vi "Router - Initial Handshaking.vi"(8 "error in (no error)":errorcluster, 11 "Router Data In":T1) -> (0 "error out":errorcluster, 3 "Router Data Out":T1)   [LabVIEW 2016, in "PXImc Router.lvlib"]
uses:
  PXImc Router.lvlib
  Controls/Router - Configuration.ctl
  Controls/Router/Node Block R-W Properties.ctl
  Controls/Router/Block Properties.ctl
  Controls/Router/Router - PXImc Properties.ctl
  Controls/Router/Router - PXImc Card Properties.ctl
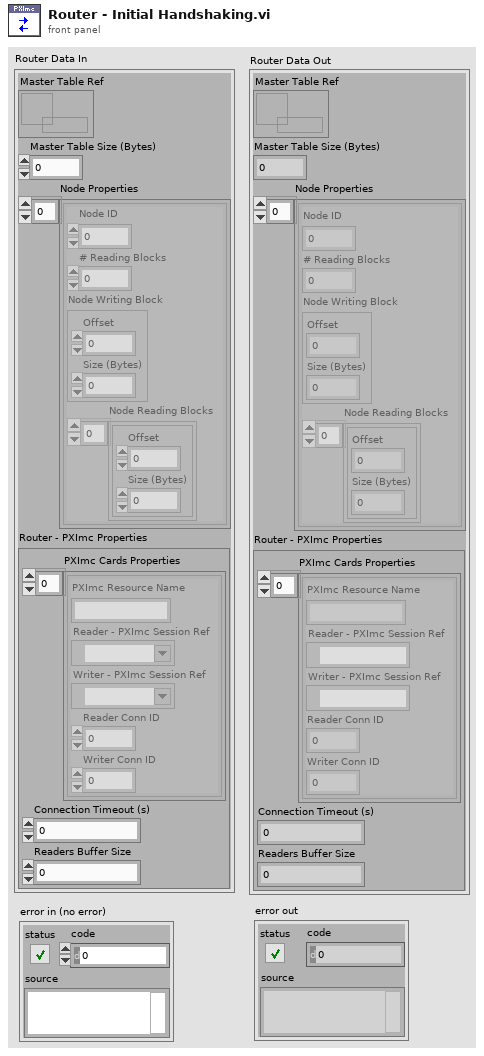
[diagram p1: front panel]
types:
  T1 = typedef "PXImc Router.lvlib/Router - Configuration.ctl" = cluster{"Master Table Ref":refnum<data-value>, "Master Table Size (Bytes)":u32, "Node Properties":T2[], "Router - PXImc Properties":T4}
  T2 = typedef "PXImc Router.lvlib/Node Block R-W Properties.ctl" = cluster{"Node ID":u32, "# Reading Blocks":u32, "Node Writing Block":T3, "Node Reading Blocks":T3[]}
  T3 = typedef "PXImc Router.lvlib/Block Properties.ctl" = cluster{"Offset":u32, "Size (Bytes)":u32}
  T4 = typedef "PXImc Router.lvlib/Router - PXImc Properties.ctl" = cluster{"PXImc Cards Properties":T5[], "Connection Timeout (s)":dbl, "Readers Buffer Size":u64}
  T5 = typedef "PXImc Router.lvlib/Router - PXImc Card Properties.ctl" = cluster{"PXImc Resource Name":string, "Reader - PXImc Session Ref":refnum<k21>, "Writer - PXImc Session Ref":refnum<k21>, "Reader Conn ID":u16, "Writer Conn ID":u16}
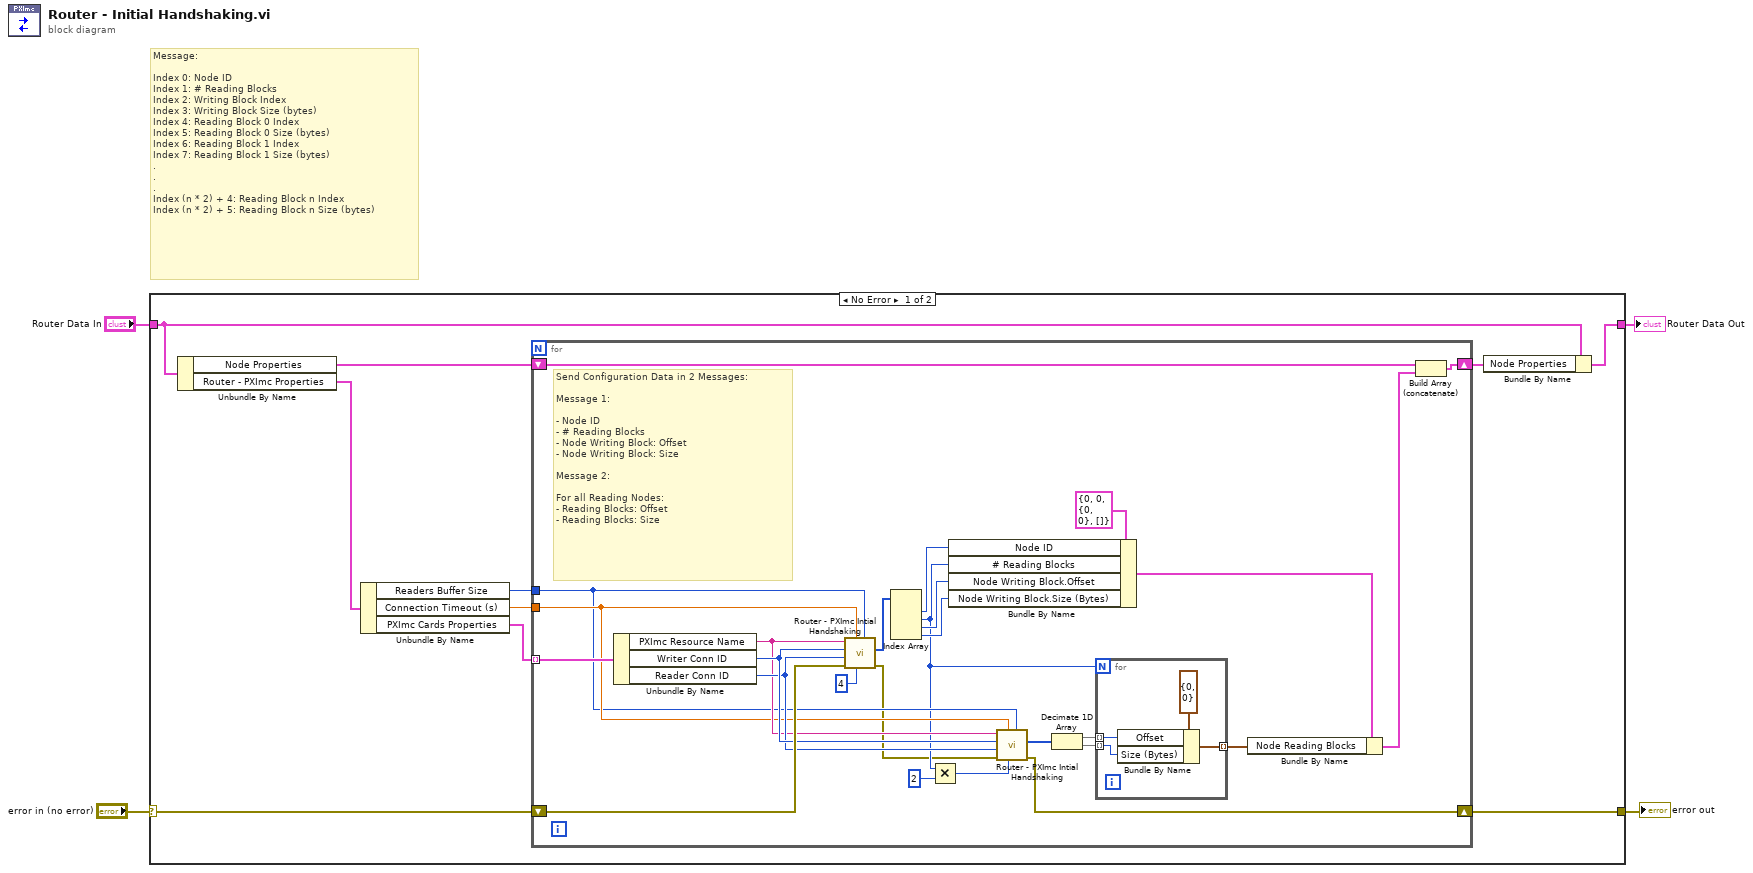
[diagram p0: block diagram]
diagram:
  # "Message:\n\nIndex 0: Node ID\nIndex 1: # Reading Blocks\nIndex 2: Writing Block Index\nIndex 3: Writing Block Size (bytes)\nIndex 4: Reading Block 0 Index\nIndex 5: Reading Block 0 Size (bytes)\nIndex 6: Reading Block 1 Index\nIndex 7: Reading Block 1 Size (bytes)\n.\n.\n.\nIndex (n * 2) + 4: Reading Block n Index\nIndex (n * 2) + 5: Reading Block n Size (bytes)"
  n1 = case shown="No Error" "error in (no error)" {
    selector: "error in (no error)" -> [w14 w46]
    tunnel: [w13 w46] -> w3
    tunnel: "Router Data In" -> [w7 w45]
    tunnel: [w6 w45] -> w1
    frame No Error {
      n2 = Unbundle By Name(w7) -> ("Node Properties"=w9:T2[], "Router - PXImc Properties"=w8:T4)
      n3 = Unbundle By Name(w8) -> ("Readers Buffer Size"=w10:u64, "Connection Timeout (s)"=w11:dbl, "PXImc Cards Properties"=w12:T5[])
      n4 = for {
        shift-right: [w19] -> w13
        shift-left: w14 -> [w34]
        tunnel: w12 -> [w39] mode=indexing
        tunnel: w11 -> [w28]
        tunnel: w10 -> [w27]
        shift-right: [w16] -> w5
        shift-left: w9 -> [w15]
        # "Send Configuration Data in 2 Messages:\n\nMessage 1:\n\n- Node ID\n- # Reading Blocks\n- Node Writing Block: Offset\n- Node Writing Block: Size\n\nMessage 2:\n\nFor all Reading Nodes: \n- Reading Blocks: Offset\n- Reading Blocks: Size"
        n5 = Unbundle By Name(w39) -> ("PXImc Resource Name"=w29:string, "Writer Conn ID"=w31:u16, "Reader Conn ID"=w30:u16)
        n6 = call "Router - PXImc Intial Handshaking.vi"("Reader Buffer Size In"=w27, "# Elements to Read"=4, "Connection Timeout (s)"=w28, "error in (no error)"=w34, "Reader Conn ID"=w30, "Writer Conn ID"=w31, "Resource Name In"=w29) -> ("error out"=w20:errorcluster, "Data Out"=w38:u32[])  [unwired: 3 in]
        n7 = Index Array(array=w38) -> (element #1=w37:u32, element #2=w25:u32, element #3=w36:u32, element #4=w35:u32)  [unwired: 4 in]
        n8 = Multiply(x=w25, y=u32 2) -> (x*y=w32:u32)
        n9 = Bundle By Name(cluster=T2 {"Node ID"=0, "# Reading Blocks"=0, "Node Writing Block"={"Offset"=0, "Size (Bytes)"=0}, "Node Reading Blocks"=[]} ("element"), "Node ID"=w37, "# Reading Blocks"=w25, "Node Writing Block.Offset"=w36, "Node Writing Block.Size (Bytes)"=w35) -> (w26:T2)
        n10 = call "Router - PXImc Intial Handshaking.vi"("Reader Buffer Size In"=w27, "# Elements to Read"=w32, "Connection Timeout (s)"=w28, "error in (no error)"=w20, "Reader Conn ID"=w30, "Writer Conn ID"=w31, "Resource Name In"=w29) -> ("error out"=w19:errorcluster, "Data Out"=w23:u32[])  [unwired: 3 in]
        n11 = Decimate 1D Array(w23) -> (w21:u32[], w22:u32[])
        n12 = for {
          N: w25 -> [_]
          tunnel: [w43] -> w24 mode=indexing
          tunnel: w22 -> [w41] mode=indexing
          tunnel: w21 -> [w42] mode=indexing
          n13 = Bundle By Name(cluster=T3 {"Offset"=0, "Size (Bytes)"=0} ("Node Writing Block"), "Offset"=w42, "Size (Bytes)"=w41) -> (w43:T3)
        }
        n14 = Bundle By Name(cluster=w26, "Node Reading Blocks"=w24) -> (w17:T2)
        n15 = Build Array (concatenate)(w15, w17) -> (w16:T2[])
      }
      n16 = Bundle By Name(cluster=w7, "Node Properties"=w5) -> (w6:T1)
    }
    frame Error {
    }
  }
  "error out" <- w3
  "Router Data Out" <- w1
